vi "Update Water Level.vi"(8 "error in (no error)":errorcluster, 10 "Water Level":dbl, 11 "Cooler UI in":refnum<class "Live User Controller.lvclass">) -> (0 "error out":errorcluster, 3 "Cooler UI out":refnum<class "Live User Controller.lvclass">)   [LabVIEW 2025, in "Live User Controller.lvclass"]
doc: "Update the user interface to show the water level."
uses:
  Live User Controller.lvclass
  Live User Controller.lvclass/Live User Controller.ctl
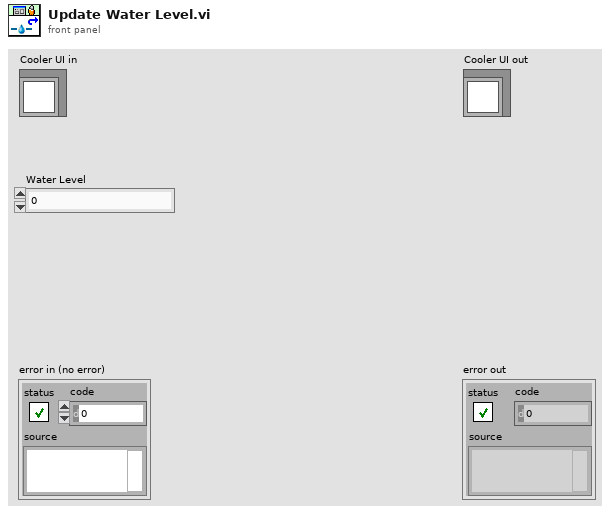
[diagram p1: front panel]
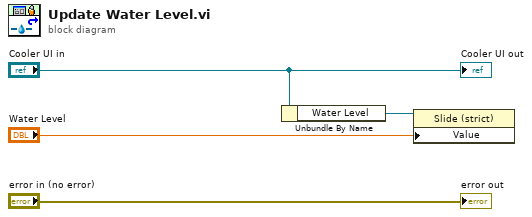
[diagram p0: block diagram]
diagram:
  n1 = Unbundle By Name("Cooler UI in") -> ("Water Level"=w1:refnum<vi>)
  n2 = property class="Slide (strict)"(reference=w1, "Value"="Water Level") -> ()  [unwired: 1 in, 2 out]
  "error out" <- "error in (no error)"
  "Cooler UI out" <- "Cooler UI in"
